vi "Save.vi"(8 "error in (no error)":errorcluster, 10 "Resampling Array":i32[](array[numeric]), 11 "DAQ Class in":refnum<class "DAQ Class.lvclass">) -> (0 "error out":errorcluster, 3 "DAQ Class out":refnum<class "DAQ Class.lvclass">)   [LabVIEW 2015, in "DAQ Class.lvclass"]
uses:
  DAQ Class.lvclass
  DAQ Class.lvclass/DAQ Class.ctl
  <vilib>/Utility/config.llb/Write Key (Double).vi
  <vilib>/Utility/config.llb/Write Key (I32).vi
  <vilib>/Utility/config.llb/Write Key (U32).vi
  <vilib>/Utility/config.llb/NI_LVConfig.lvlib
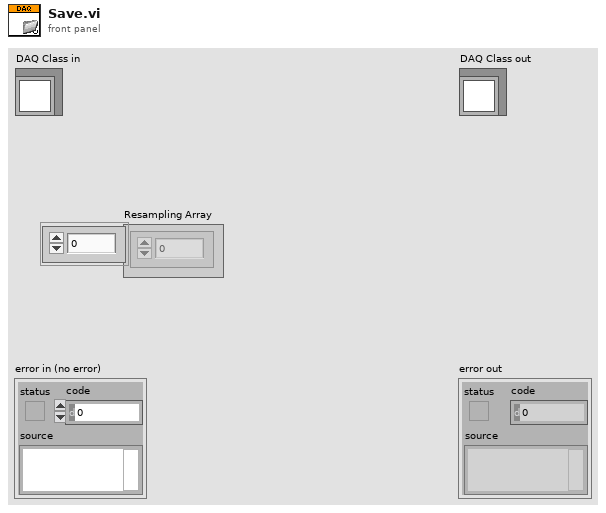
[diagram p1: front panel]
types:
  T1 = typedef "DAQ Class.lvclass/DAQ Parameters.ctl" = cluster{"Points Per A-Scan":u32, "A-Scans Per B-Scan":u32, "Number of B-Scans":u32, "B-Scans Per Transfer":u32, "Trigger Voltage":sgl, "Trigger Source":T2, "Trigger Slope":T3, "Channel":T4, "Clock":T5, "Bits per Sample":dbl, "Range":dbl, "Start Trim":u32, "Stop Trim":u32}
  T2 = typedef "DAQ Class.lvclass/Trigger Source.ctl" = enum16{"External", "Channel A", "Channel B"}
  T3 = typedef "DAQ Class.lvclass/Trigger Slope.ctl" = enum16{"Rising", "Falling"}
  T4 = typedef "OCT DAQ Channel Data Type.ctl" = enum16{"Channel 1", "Channel 2", "Channel 1 and 2"}
  T5 = typedef "DAQ Class.lvclass/Clock Control.ctl" = enum16{"Internal Clock", "External Clock"}
  T6 = typedef "NI_LVConfig.lvlib/Config Data RefNum.ctl" = refnum<k1>
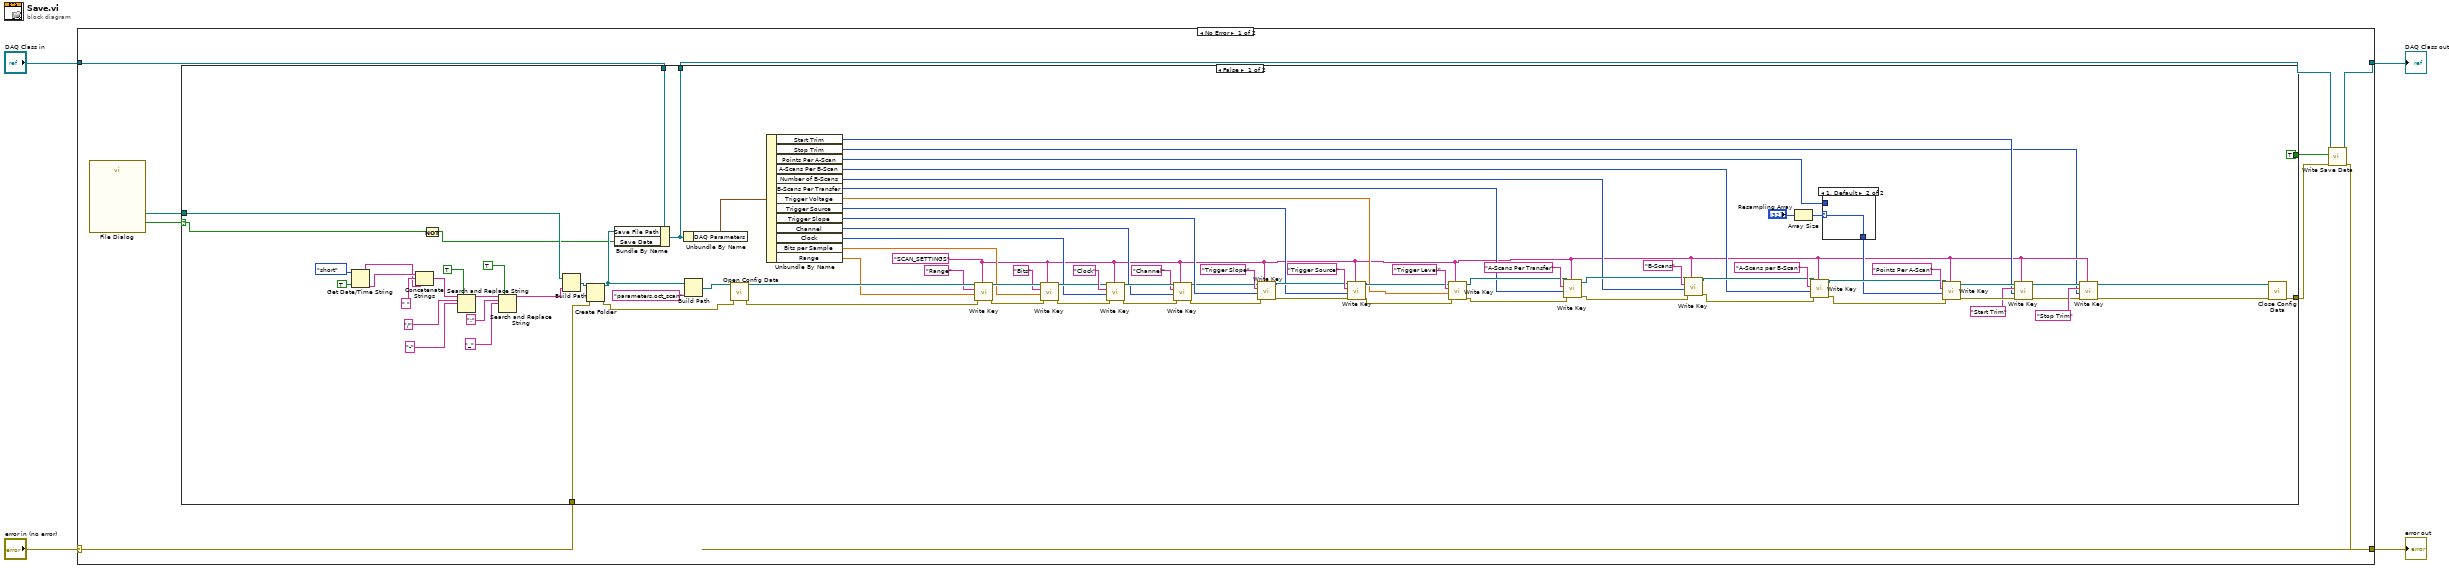
[diagram p0: block diagram]
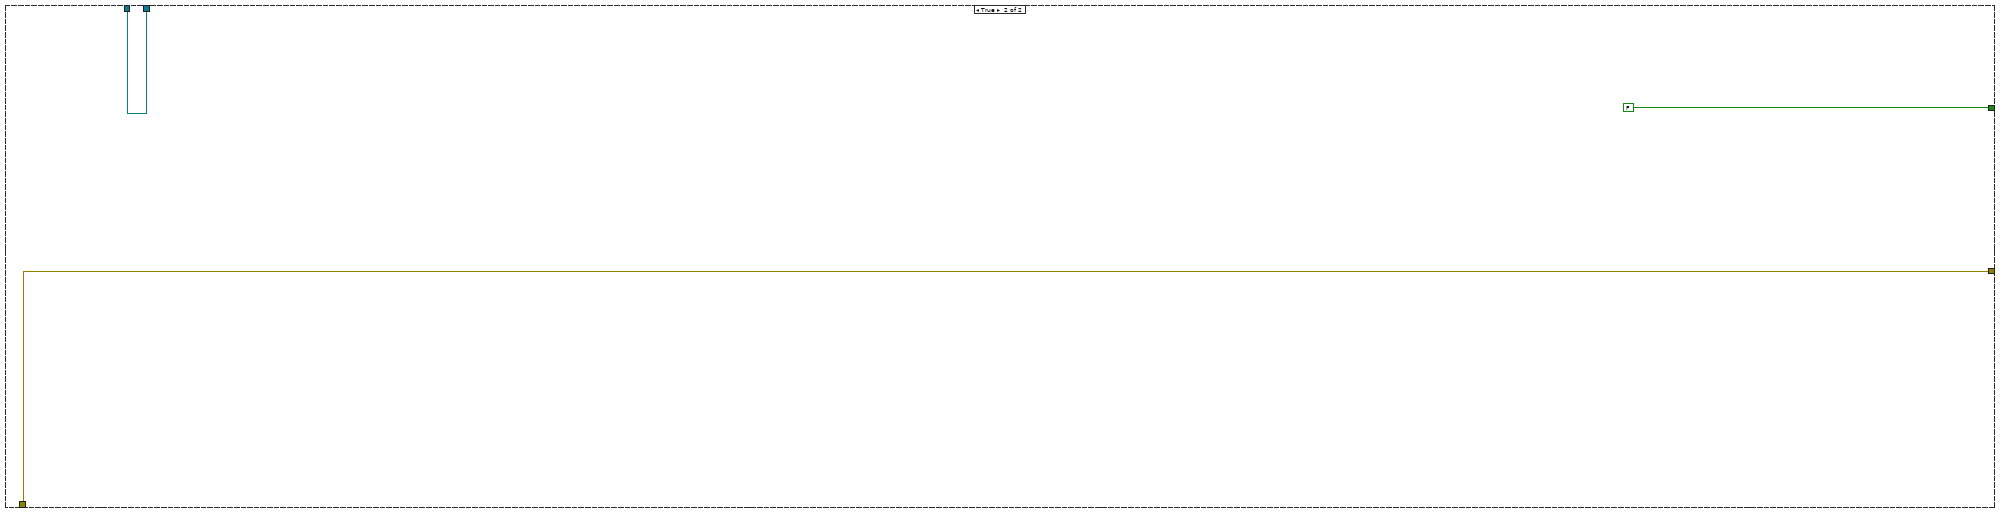
[diagram p3: hidden frame]
diagram:
  n1 = case shown="No Error" "error in (no error)" {
    selector: "error in (no error)" -> [w12 w106]
    tunnel: [w9 w106] -> w3
    tunnel: [w8 w105] -> w1
    tunnel: "DAQ Class in" -> [w11 w105]
    frame No Error {
      n2 = call "File Dialog"() -> ("selected path"=w13:path, "cancelled"=w5:bool)  [unwired: 12 in, 2 out]
      n3 = case shown="False" w5 {
        selector: w5 -> [w26 _]
        tunnel: w13 -> [w95 _]
        tunnel: w12 -> [w84 w102]
        tunnel: w11 -> [w74 w104]
        tunnel: [w30 w102] -> w10
        tunnel: [TRUE ("Save Data") FALSE ("Save Data")] -> w7
        tunnel: [w28 w104] -> w6
        frame False {
          w17 = "SCAN_SETTINGS" ("section")
          n4 = Get Date/Time String(date format (0)=enum16{"short", "long", "abbreviated"}."short", want seconds? (F)=TRUE) -> (date string=w97:string, time string=w98:string)  [unwired: 1 in]
          n5 = Concatenate Strings(w98, " " ("string"), w97) -> (w93:string)
          n6 = Not(x=w26) -> (.not. x?=w25:bool)
          n7 = Search and Replace String(replace all?=TRUE ("replace all? (F)"), input string=w93, search string="/", replace string="-" ("search string")) -> (result string=w90:string)  [unwired: 4 in, 3 out]
          n8 = Search and Replace String(replace all?=TRUE ("replace all? (F)"), input string=w90, search string=":", replace string="_" ("search string")) -> (result string=w89:string)  [unwired: 4 in, 3 out]
          n9 = Build Path(base path=w95, name or relative path=w89) -> (appended path=w85:path)
          n10 = Create Folder(path (use dialog)=w85, error in=w84) -> (created path=w83:path, error out=w80:errorcluster)  [unwired: 1 in, 1 out]
          n11 = Bundle By Name(cluster=w74, "Save File Path"=w83, "Save Data"=w25) -> (w28:refnum<class "DAQ Class.lvclass">)
          n12 = Unbundle By Name(w28) -> ("DAQ Parameters"=w77:T1)
          n13 = Build Path(base path=w83, name or relative path="parameters.oct_scan") -> (appended path=w81:path)
          n14 = call <vilib>:"Open Config Data.vi"("error in (no error)"=w80, "configuration file path"=w81) -> ("error out"=w78:errorcluster, "refnum"=w79:T6)  [unwired: 7 in, 1 out]
          n15 = Unbundle By Name(w77) -> ("Start Trim"=w21:u32, "Stop Trim"=w16:u32, "Points Per A-Scan"=w32:u32, "A-Scans Per B-Scan"=w39:u32, "Number of B-Scans"=w43:u32, "B-Scans Per Transfer"=w47:u32, "Trigger Voltage"=w51:sgl, "Trigger Source"=w55:T2, "Trigger Slope"=w60:T3, "Channel"=w63:T4, "Clock"=w67:T5, "Bits per Sample"=w71:dbl, "Range"=w76:dbl)
          n16 = call-poly <vilib>:"Write Key.vi"("section"=w17, "error in (no error)"=w78, "value"=w76, "key"="Range", "refnum"=w79) -> ("error out"=w35:errorcluster, "refnum out"=w73:T6)  [unwired: 4 in, 1 out]
          n17 = call-poly <vilib>:"Write Key.vi"("section"=w17, "error in (no error)"=w35, "value"=w71, "key"="Bits", "refnum"=w73) -> ("error out"=w69:errorcluster, "refnum out"=w68:T6)  [unwired: 4 in, 1 out]
          n18 = call-poly <vilib>:"Write Key.vi"("section"=w17, "error in (no error)"=w69, "value"=w67, "key"="Clock", "refnum"=w68) -> ("error out"=w65:errorcluster, "refnum out"=w66:T6)  [unwired: 4 in, 1 out]
          n19 = call-poly <vilib>:"Write Key.vi"("section"=w17, "error in (no error)"=w65, "value"=w63, "key"="Channel", "refnum"=w66) -> ("error out"=w61:errorcluster, "refnum out"=w59:T6)  [unwired: 4 in, 1 out]
          n20 = call-poly <vilib>:"Write Key.vi"("section"=w17, "error in (no error)"=w61, "value"=w60, "key"="Trigger Slope", "refnum"=w59) -> ("error out"=w57:errorcluster, "refnum out"=w56:T6)  [unwired: 4 in, 1 out]
          n21 = call-poly <vilib>:"Write Key.vi"("section"=w17, "error in (no error)"=w57, "value"=w55, "key"="Trigger Source", "refnum"=w56) -> ("error out"=w53:errorcluster, "refnum out"=w52:T6)  [unwired: 4 in, 1 out]
          n22 = call-poly <vilib>:"Write Key.vi"("section"=w17, "error in (no error)"=w53, "value"=w51, "key"="Trigger Level", "refnum"=w52) -> ("error out"=w49:errorcluster, "refnum out"=w48:T6)  [unwired: 4 in, 1 out]
          n23 = call-poly <vilib>:"Write Key.vi"("section"=w17, "error in (no error)"=w49, "value"=w47, "key"="A-Scans Per Transfer", "refnum"=w48) -> ("error out"=w45:errorcluster, "refnum out"=w44:T6)  [unwired: 4 in, 1 out]
          n24 = call-poly <vilib>:"Write Key.vi"("section"=w17, "error in (no error)"=w45, "value"=w43, "key"="B-Scans", "refnum"=w44) -> ("error out"=w40:errorcluster, "refnum out"=w41:T6)  [unwired: 4 in, 1 out]
          n25 = Array Size(array="Resampling Array") -> (size(s)=w33:i32)
          n26 = call-poly <vilib>:"Write Key.vi"("section"=w17, "error in (no error)"=w40, "value"=w39, "key"="A-Scans per B-Scan", "refnum"=w41) -> ("error out"=w36:errorcluster, "refnum out"=w37:T6)  [unwired: 4 in, 1 out]
          n27 = case shown="1, Default" w33 {
            selector: w33 -> [_ w101]
            tunnel: w32 -> [w100 _]
            tunnel: [w100 w101] -> w31
            frame 0 {
            }
            frame 1, Default {
            }
          }
          n28 = call-poly <vilib>:"Write Key.vi"("section"=w17, "error in (no error)"=w36, "value"=w31, "key"="Points Per A-Scan", "refnum"=w37) -> ("error out"=w23:errorcluster, "refnum out"=w24:T6)  [unwired: 4 in, 1 out]
          n29 = call-poly <vilib>:"Write Key.vi"("section"=w17, "error in (no error)"=w23, "value"=w21, "key"="Start Trim", "refnum"=w24) -> ("error out"=w19:errorcluster, "refnum out"=w18:T6)  [unwired: 4 in, 1 out]
          n30 = call-poly <vilib>:"Write Key.vi"("section"=w17, "error in (no error)"=w19, "value"=w16, "key"="Stop Trim", "refnum"=w18) -> ("error out"=w14:errorcluster, "refnum out"=w15:T6)  [unwired: 4 in, 1 out]
          n31 = call <vilib>:"Close Config Data.vi"("error in (no error)"=w14, "refnum"=w15) -> ("error out"=w30:errorcluster)  [unwired: 8 in, 1 out]
        }
        frame True {
        }
      }
      n32 = call-dynamic "Write Save Data.vi"("error in (no error)"=w10, "Save Data"=w7, "DAQ Class in"=w6) -> ("error out"=w9:errorcluster, "DAQ Class out"=w8:refnum<class "DAQ Class.lvclass">)  [unwired: 7 in]
    }
    frame Error {
    }
  }
  "error out" <- w3
  "DAQ Class out" <- w1
